vi "rx.vi"() -> ()   [LabVIEW 2016]
uses:
  <vilib>/Instr/_visa.llb/VISA Configure Serial Port (Instr).vi
panel:
  in  "Tab Control":enum32{"Raw", "Diff"}(tab)
  out "Raw":i32(graph)=220
  out "Diff":i16(graph)
  in  "VISA resource name":refnum<visa-resource-name>="COM1"
  out "error out":errorcluster
  in  "stop":bool
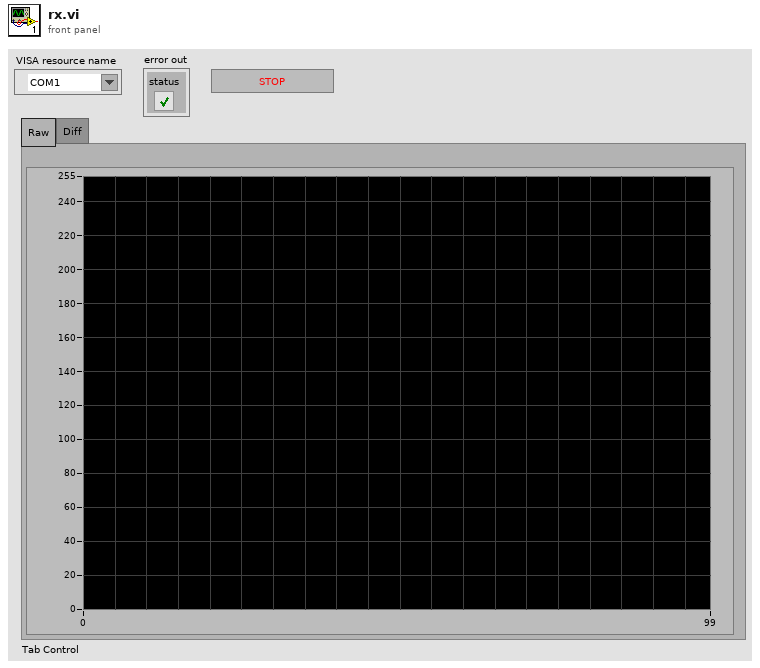
[diagram p1: front panel]
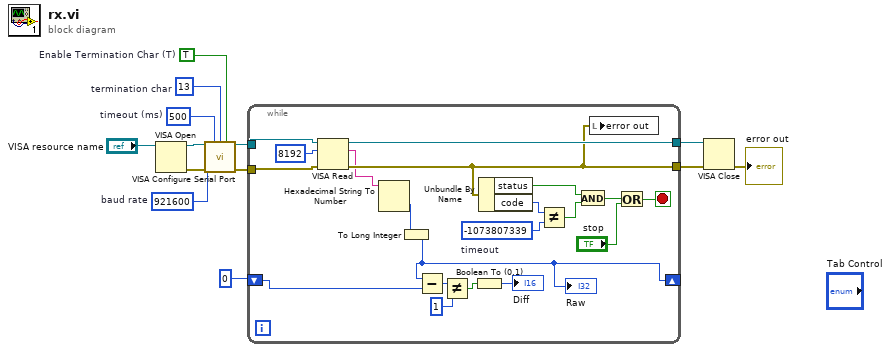
[diagram p0: block diagram]
diagram:
  w2 = u32 921600  # baud rate
  w3 = u32 500  # timeout (ms)
  w9 = TRUE  # Enable Termination Char (T)
  w10 = u8 13  # termination char
  n1 = VISA Open(VISA resource name="VISA resource name") -> (VISA resource name=w12:refnum<visa-resource-name>, error out=w13:errorcluster)  [unwired: 4 in]
  n2 = call-poly "VISA Configure Serial Port"("VISA resource name"=w12, "timeout (10sec)"=w3, "termination char\n(0xA = '\\n' = LF)"=w10, "Enable Termination\nChar (T)"=w9, "baud rate (9600)"=w2, "error in (no error)"=w13) -> ("VISA resource name out"=w6:refnum<visa-resource-name>, "error out"=w5:errorcluster)  [unwired: 8 in]
  n3 = while {
    tunnel: w6 -> [w23]
    tunnel: [w33] -> w8
    tunnel: w5 -> [w22]
    tunnel: [w31] -> w7
    shift-right: [w18] -> _
    shift-left: 0 ("Measurement") -> [w20]
    stop <- w25 stop-if-true
    w29 = -1073807339  # timeout
    n4 = VISA Read(VISA resource name=w23, byte count=u32 8192, error in (no error)=w22) -> (VISA resource name out=w33:refnum<visa-resource-name>, read buffer=w21:string, error out=w31:errorcluster)  [unwired: 1 out]
    n5 = Hexadecimal String To Number(string=w21) -> (number=w19:u32)  [unwired: 2 in, 1 out]
    n6 = To Long Integer(number=w19) -> (32bit integer=w18:i32)
    "Raw" <- w18
    n7 = Subtract(x=w18, y=w20) -> (x-y=w16:i32)
    n8 = Not Equal?(x=w16, y=1) -> (x != y?=w14:bool)
    n9 = Boolean To (0,1)(Boolean=w14) -> (0, 1=→"Diff":i16)
    n10 = Unbundle By Name(w31) -> ("status"=w27:bool, "code"=w30:i32)
    n11 = Not Equal?(x=w30, y=w29) -> (x != y?=w28:bool)
    n12 = And(x=w27, y=w28) -> (x .and. y?=w26:bool)
    n13 = local write "error out"(w31) -> ()
    n14 = Or(x=w26, y="stop") -> (x .or. y?=w25:bool)
  }
  n15 = VISA Close(VISA resource name=w8, error in (no error)=w7) -> (error out=→"error out":errorcluster)
